vi "Read add enable channel.vi"(8 "error in (no error)":errorcluster, 11 "TDMS datalogger configuration in":refnum<class "TDMS datalogger configuration.lvclass">) -> (0 "error out":errorcluster, 2 "add enable channel":bool, 3 "TDMS datalogger configuration out":refnum<class "TDMS datalogger configuration.lvclass">)   [LabVIEW 2015, in "TDMS datalogger configuration.lvclass"]
uses:
  TDMS datalogger configuration.lvclass
  TDMS datalogger configuration.lvclass/TDMS datalogger configuration.ctl
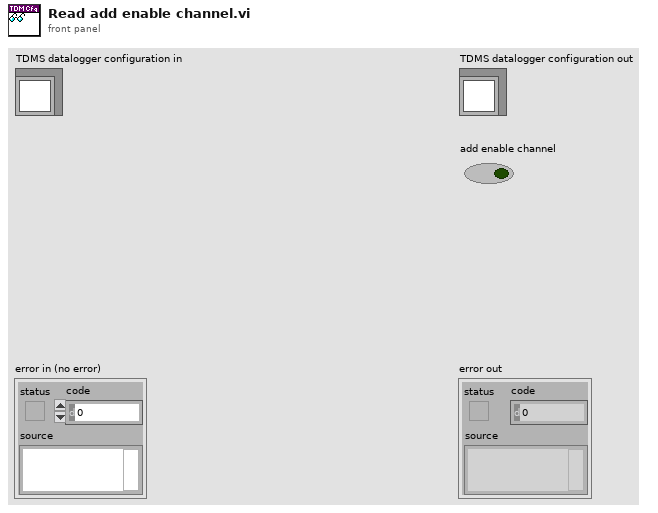
[diagram p1: front panel]
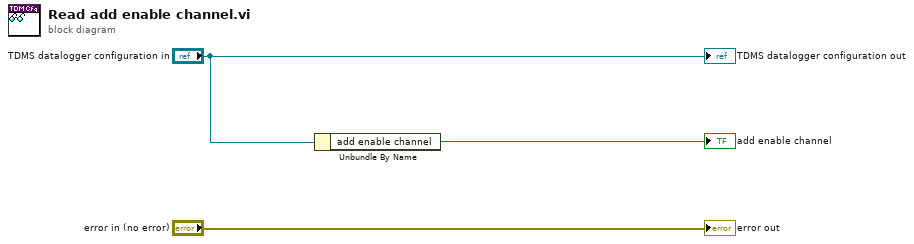
[diagram p0: block diagram]
diagram:
  n1 = Unbundle By Name("TDMS datalogger configuration in") -> ("add enable channel"=→"add enable channel":bool)
  "error out" <- "error in (no error)"
  "TDMS datalogger configuration out" <- "TDMS datalogger configuration in"
